vi "FRCts20_WebMethods_ReadData_PUT_Comment.vi"(8 "error in (no error)":errorcluster, 10 "Request":T1, 11 "httpRequestID":u32) -> (0 "error out":errorcluster, 2 "Request 2":T1, 3 "httpRequestID out":u32)   [LabVIEW 2014, in "FRCts20_WebMethods.lvlib"]
uses:
  FRCts20_WebMethods.lvlib
  <vilib>/wsapi/NI_WebServices.lvlib
  Backend/source/VI Source/FRCts20_Backend_API/FRCts20_Backend_API_Status.ctl
  Backend/source/VI Source/FRCts20_Backend_API/FRCts20_Backend_API.lvlib
  Web Method Public Interface/FRCts20_WebMethods_ctl_request.ctl
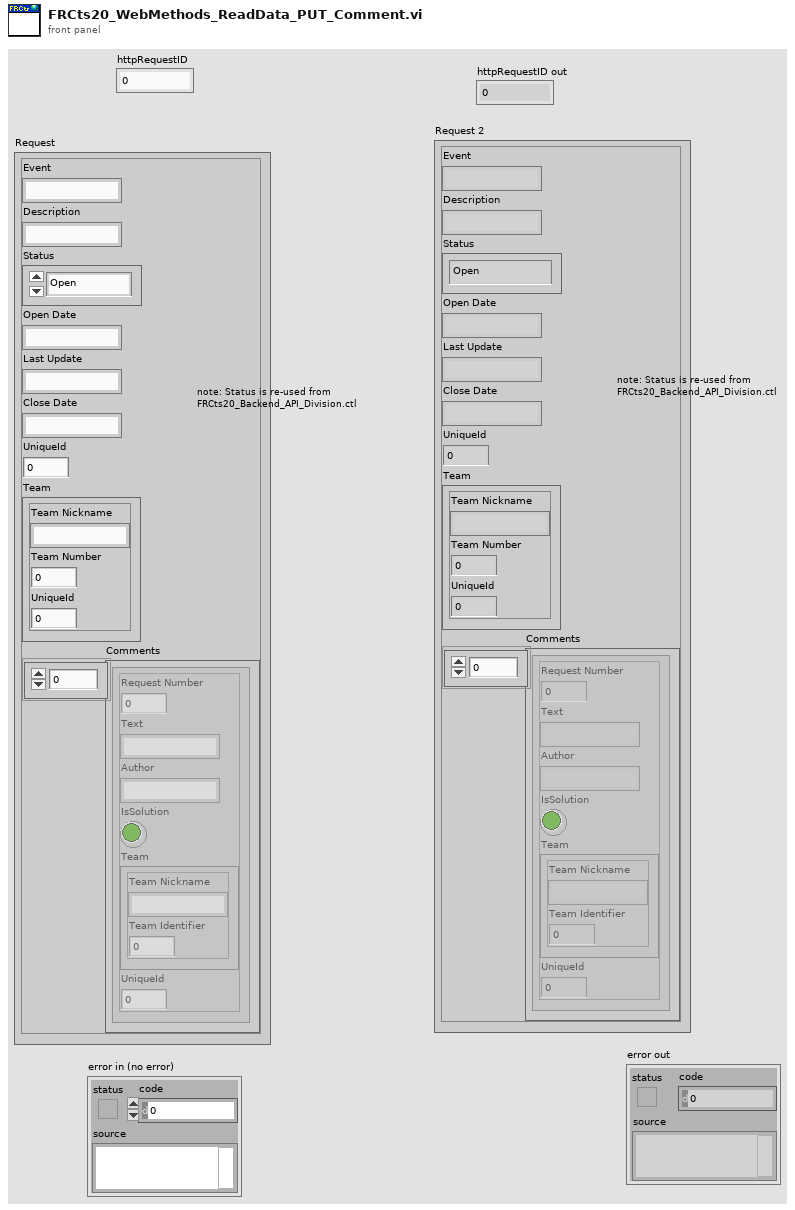
[diagram p1: front panel]
types:
  T1 = typedef "FRCts20_WebMethods.lvlib/FRCts20_WebMethods_ctl_request.ctl" = cluster{"Event":string, "Description":string, "Status":T2, "Open Date":string, "Last Update":string, "Close Date":string, "UniqueId":i32, "Team":cluster{"Team Nickname":string, "Team Number ":i32, "UniqueId":i32}, "Comments":cluster{"Request Number":dbl, "Text":string, "Author":string, "IsSolution":bool, "Team":cluster{"Team Nickname":string, "Team Identifier ":dbl}, "UniqueId":i32}[]}
  T2 = typedef "FRCts20_Backend_API.lvlib/FRCts20_Backend_API_Status.ctl" = enum16{"Open", "In Work", "Closed"}
  T3 = typedef "FRCts20_WebMethods.lvlib/FRCts20_WebMethods_ctl_returntype.ctl" = string
  T4 = cluster{"Request Number":dbl, "Text":string, "Author":string, "IsSolution":bool, "Team":cluster{"Team Nickname":string, "Team Identifier ":dbl}, "UniqueId":i32}[]
  T5 = cluster{"Request Number":dbl, "Text":string, "Author":string, "IsSolution":bool, "Team":cluster{"Team Nickname":string, "Team Identifier ":dbl}, "UniqueId":i32}
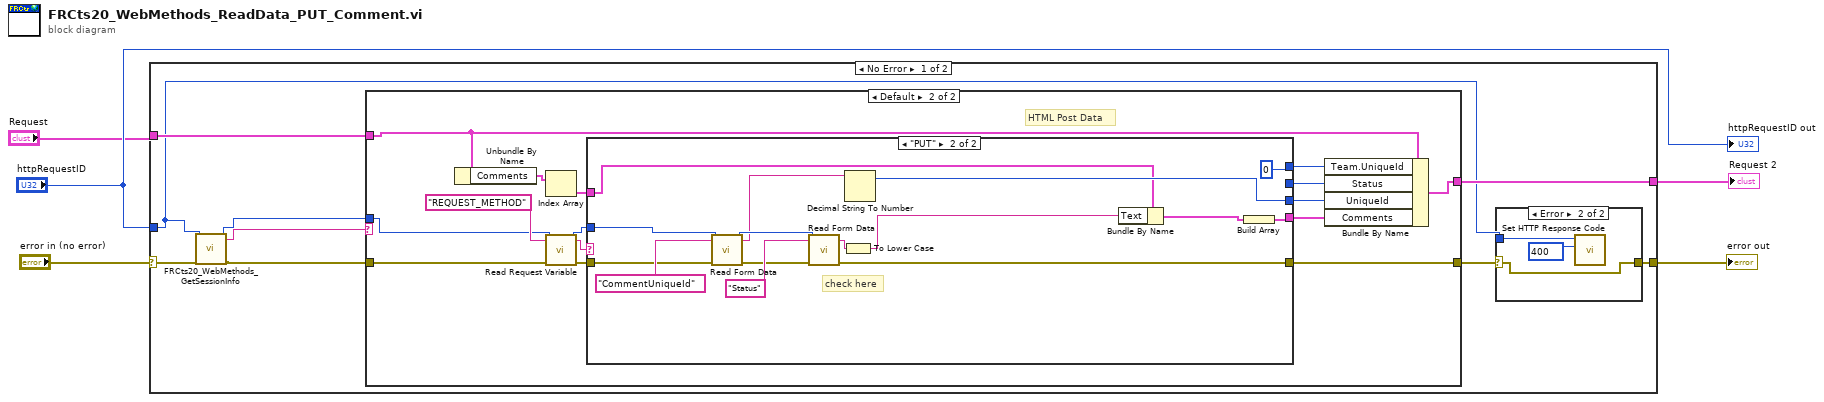
[diagram p0: block diagram]
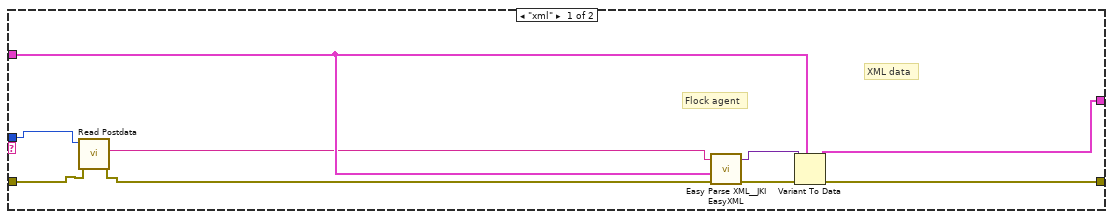
[diagram p3: hidden frame]
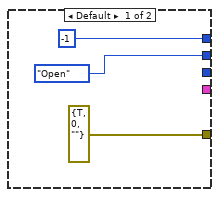
[diagram p4: hidden frame]
diagram:
  n1 = case shown="No Error" "error in (no error)" {
    selector: "error in (no error)" -> [w9 w62]
    tunnel: "httpRequestID" -> [w8 _]
    tunnel: "Request" -> [w14 w61]
    tunnel: [w11 w62] -> w4
    tunnel: [w12 w61] -> w1
    frame No Error {
      n2 = call "FRCts20_WebMethods_GetSessionInfo.vi"("error in"=w9, "httpRequestID"=w8) -> ("error out"=w10:errorcluster, "Return Type"=w7:T3, "httpRequestID out"=w6:u32)  [unwired: 7 in]
      n3 = case shown="Default" w7 {
        tunnel: w10 -> [w22 w39]
        tunnel: w14 -> [w25 w32]
        tunnel: [w24 w42] -> w13
        tunnel: [w23 w41] -> w12
        tunnel: w6 -> [w19 w34]
        frame "xml" {
          # "Flock agent"
          # "XML data"
          n4 = call <vilib>:"Read Postdata.vi"("error in (no error)"=w22, "httpRequestID"=w19) -> ("error out"=w21:errorcluster, "postdata"=w20:string)  [unwired: 7 in, 1 out]
          n5 = call <vilib>:"Easy Parse XML__JKI EasyXML.vi"("error in (no error)"=w21, "LabVIEW Data (Type)"=w25, "XML String"=w20) -> ("error out"=w27:errorcluster, "LabVIEW Data"=w26:variant)  [unwired: 7 in]
          n6 = Variant To Data(error in=w27, type=w25, Variant=w26) -> (data=w23:T1, error out=w24:errorcluster)
        }
        frame Default {
          # "HTML Post Data"
          n7 = Unbundle By Name(w32) -> ("Comments"=w31:T4)
          n8 = Index Array(array=w31) -> (element=w30:T5)  [unwired: 1 in]
          n9 = call <vilib>:"Read Request Variable.vi"("error in (no error)"=w39, "variable name"="REQUEST_METHOD", "httpRequestID"=w34) -> ("error out"=w38:errorcluster, "value"=w37:string, "httpRequestID out"=w36:u32)  [unwired: 6 in]
          n10 = case shown="\"PUT\"" w37 {
            tunnel: [errorcluster {"status"=TRUE, "code"=0, "source"=""} ("error out") w53] -> w42
            tunnel: [-1 0] -> w35
            tunnel: w38 -> [_ w55]
            tunnel: w36 -> [_ w54]
            tunnel: [_ w50] -> w33
            tunnel: w30 -> [_ w49]
            tunnel: [_ w48] -> w29
            tunnel: [FRCts20_Backend_API_Status."Open" ("Status") _] -> w28
            frame Default {
            }
            frame "PUT" {
              # "check here"
              n11 = call <vilib>:"Read Form Data.vi"("error in (no error)"=w55, "key"="CommentUniqueId", "httpRequestID"=w54) -> ("error out"=w57:errorcluster, "value"=w51:string, "httpRequestID out"=w56:u32)  [unwired: 5 in, 1 out]
              n12 = call <vilib>:"Read Form Data.vi"("error in (no error)"=w57, "key"="Status", "httpRequestID"=w56) -> ("error out"=w53:errorcluster, "value"=w59:string)  [unwired: 5 in, 2 out]
              n13 = To Lower Case(string=w59) -> (all lower case string=w46:string)
              n14 = Decimal String To Number(string=w51) -> (offset past number=w50:i32)  [unwired: 2 in, 1 out]
              n15 = Bundle By Name(cluster=w49, "Text"=w46) -> (w47:T5)
              n16 = Build Array(w47) -> (w48:T4)
            }
          }
          n17 = Bundle By Name(cluster=w32, "Team.UniqueId"=w35, "Status"=w28, "UniqueId"=w33, "Comments"=w29) -> (w41:T1)
        }
      }
      n18 = case shown="Error" w13 {
        selector: w13 -> [w15 w16]
        tunnel: [w15 w16] -> w11
        tunnel: w8 -> [_ w17]
        frame No Error {
        }
        frame Error {
          w18 = 400 items=["100"=100, "101"=101, "200"=200, "201"=201, "202"=202, "203"=203, "204"=204, "205"=205, "206"=206, "300"=300, "301"=301, "302"=302, "303"=303, "304"=304, "305"=305, "306"=306, "307"=307, "400"=400, "401"=401, "402"=402, "403"=403, "404"=404, "405"=405, "406"=406, "407"=407, "408"=408, "409"=409, "410"=410, "411"=411, "412"=412, "413"=413, "414"=414, "415"=415, "416"=416, "417"=417, "500"=500, "501"=501, "502"=502, "503"=503, "504"=504, "505"=505] ("response code (200)")
          n19 = call <vilib>:"Set HTTP Response Code.vi"("response code (200)"=w18, "httpRequestID"=w17) -> ()  [unwired: 8 in, 2 out]
        }
      }
    }
    frame Error {
    }
  }
  "Request 2" <- w1
  "error out" <- w4
  "httpRequestID out" <- "httpRequestID"
